vi "LVClass_HasoData Save to file.vi"(0 "HasoData in":refnum<class "HasoData.lvclass">, 5 "HAS file path":path, 7 "session_name":string, 9 "comments":string, 11 "error in (no error)":errorcluster) -> (4 "HasoData out":refnum<class "HasoData.lvclass">, 15 "error out":errorcluster)   [LabVIEW 2020, in "HasoData.lvclass"]
doc: "Saves a HasoData object to a .has file. If file already exists, it is\noverwritten, provided that opening succeeds. If file opening fails, an\nexception is thrown.\n\n--------------------------------------------------------------------------------\n\n<B>HasoDataIn </B> : HasoData object.\n<B>HasoDataOut </B> : HasoData object.\n<B>has_file_path </B> : Absolute path to the .has file.\n<B>comments </B> : Comments.\n<B>session_name </B> : Session name.\n<B>ErrorIn </B> : Error\n<B>ErrorOut </B> : Error\n\n--------------------------------------------------------------------------------"
uses:
  HasoData.lvclass
  HasoData.lvclass/HasoData.ctl
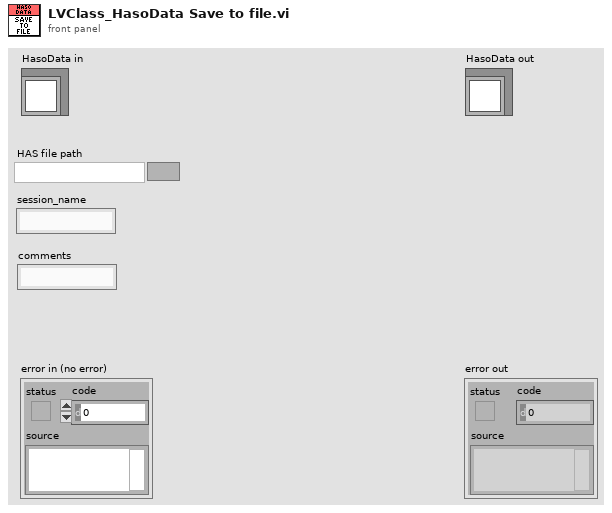
[diagram p1: front panel]
types:
  T1 = enum32{"existing file", "new file", "new or existing file", "existing dir", "new dir", "new or existing dir", "existing file (use LLBs)", "new file (use LLBs)", "new or existing file (use LLBs)", "new or existing file or directory (use LLBs)", "existing dir (use LLBs)", "new dir (use LLBs)", "new or existing dir (use LLBs)", "existing file or dir", "new file or dir", "new or existing file or dir", "existing file or dir (use LLBs)", "new file or dir (use LLBs)", "multi-select", "multi-select (use LLBs)"}
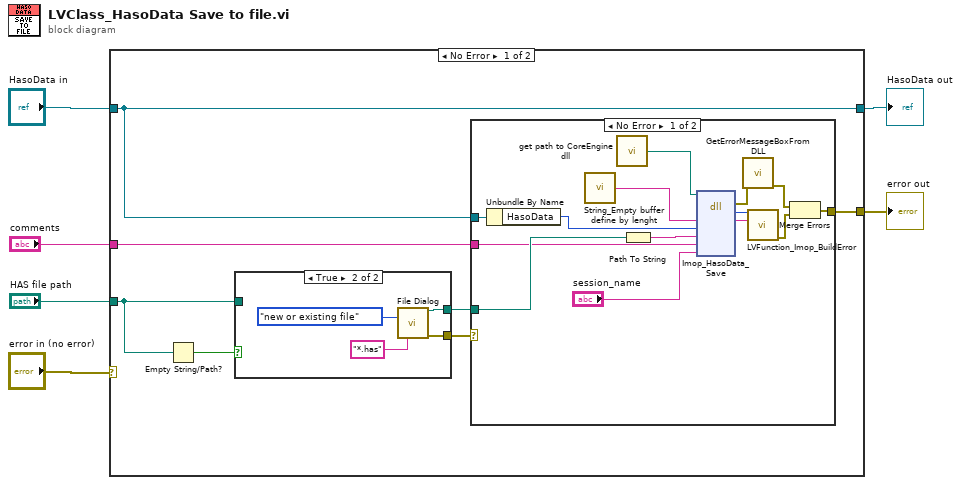
[diagram p0: block diagram]
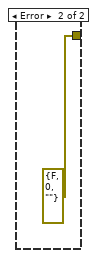
[diagram p2: hidden frame]
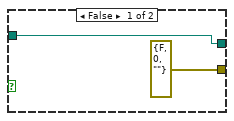
[diagram p3: hidden frame]
diagram:
  n1 = case shown="No Error" "error in (no error)" {
    selector: "error in (no error)" -> [_ w36]
    tunnel: [w13 w36] -> w3
    tunnel: [w12 w35] -> w4
    tunnel: "HasoData in" -> [w12 w35]
    tunnel: "HAS file path" -> [w10 _]
    tunnel: "comments" -> [w7 _]
    frame No Error {
      n2 = Empty String/Path?(string/path=w10) -> (empty?=w11:bool)
      n3 = case shown="True" w11 {
        tunnel: [w30 w33] -> w9
        tunnel: w10 -> [w30 _]
        tunnel: [errorcluster {"status"=FALSE, "code"=0, "source"=""} ("error out") w32] -> w8
        frame False {
        }
        frame True {
          n4 = call "File Dialog.vi"("selection mode"=T1."new or existing file", "pattern (all files)"="*.has") -> ("selected path"=w33:path, "error out"=w32:errorcluster)  [unwired: 10 in, 2 out]
        }
      }
      n5 = case shown="No Error" w8 {
        tunnel: [w16 errorcluster {"status"=FALSE, "code"=0, "source"=""} ("error out")] -> w13
        tunnel: w12 -> [w22 _]
        tunnel: w9 -> [w19 _]
        tunnel: w7 -> [w15 _]
        frame No Error {
          n6 = Unbundle By Name(w22) -> ("HasoData"=w21:i32)
          n7 = call "String_Empty buffer define by lenght.vi"() -> ("Empty buffer"=w25:string)  [unwired: 1 in]
          n8 = call "get path to CoreEngine dll.vi"() -> ("path to c_interface_vc100.dll"=w24:path)  [unwired: 12 in, 3 out]
          n9 = Path To String(path=w19) -> (string=w20:string)
          n10 = dll-call lib="D:/2_trunk/Soft_haso/ImOpCoreEngine4_LV2011/DLLs/ImopEngine4_vc100.dll" fn="Imop_HasoData_Save"(path in=w24, "message"=w25, "objet"=w21, "HasFilePath"=w20, "comments"=w15, "session_name"="session_name") -> (error out=w23:errorcluster, "return type"=w27:i32, "message"=w26:string)  [unwired: 6 in, 1 out]
          n11 = call "GetErrorMessageBoxFromDLL.vi"("error IN"=w23) -> ("error OUT"=w18:errorcluster)  [unwired: 10 in]
          n12 = call "LVFunction_Imop_BuildError.vi"("code"=w27, "String to Prepend to source (\"\")"=w26) -> ("error out"=w17:errorcluster)  [unwired: 13 in]
          n13 = Merge Errors(w18, w17) -> (w16:errorcluster)
        }
        frame Error {
        }
      }
    }
    frame Error {
    }
  }
  "error out" <- w3
  "HasoData out" <- w4
